vi "Retain Or Reset Sub Value.vi"(7 "ListBox in":refnum<vi>, 8 "error in (no error)":errorcluster, 11 "sub object":T1) -> (0 "error out":errorcluster)   [LabVIEW 2020, in "Navigation.lvlib" / "Button Manager.lvclass"]
doc: "____\nHAMPEL SOFTWARE ENGINEERING v2.6.0 (2023-12-19 10:54)"
uses:
  Button Manager.lvclass
  Sub Control.ctl
  Button Manager.lvclass/Button Manager.ctl
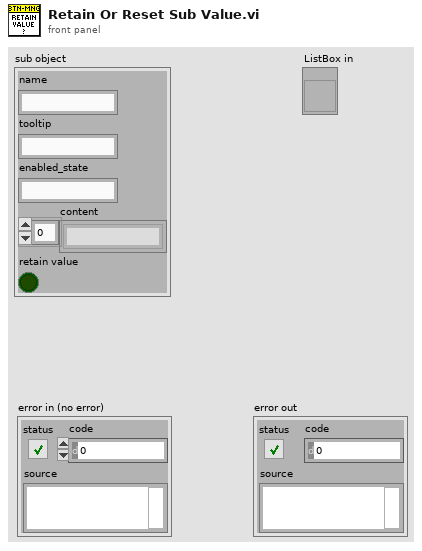
[diagram p1: front panel]
types:
  T1 = typedef "Navigation.lvlib/Button Manager.lvclass/Sub Control.ctl" = cluster{"name":string, "tooltip":string, "enabled_state":string, "content":string[], "retain value":bool}
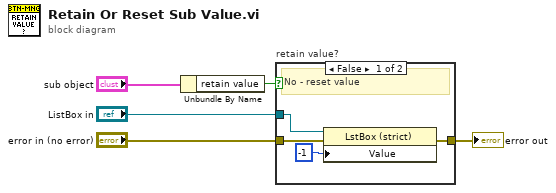
[diagram p0: block diagram]
diagram:
  n1 = Unbundle By Name("sub object") -> ("retain value"=w3:bool)
  n2 = case "retain value?" shown="False" w3 {
    tunnel: "ListBox in" -> [w9 _]
    tunnel: "error in (no error)" -> [w7 w10]
    tunnel: [w6 w10] -> w5
    frame False {
      # "No - reset value"
      n3 = property class="LstBox (strict)"(reference=w9, error in=w7, "Value"=-1) -> (error out=w6:errorcluster)  [unwired: 1 out]
    }
    frame True {
      # "Yes - do nothing"
    }
  }
  "error out" <- w5
